vi "Get JSON Config.vi"(11 "CFG Base in":refnum<class "CFG JSON.lvclass">) -> (2 "<JSON>Config>":string, 3 "CFG Base out":refnum<class "CFG JSON.lvclass">)   [LabVIEW 2023, in "HAL GOOP4.lvlib" / "CFG JSON.lvclass"]
uses:
  CFG JSON.lvclass
  CFG JSON.lvclass/CFG JSON.ctl
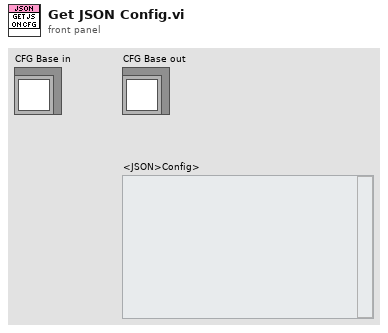
[diagram p1: front panel]
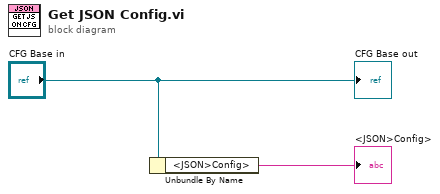
[diagram p0: block diagram]
diagram:
  n1 = Unbundle By Name("CFG Base in") -> ("<JSON>Config>"=→"<JSON>Config>":string)
  "CFG Base out" <- "CFG Base in"
